vi "FPGASwitch.vi"() -> ()   [LabVIEW 2015]
uses:
  Switch/SwitchStates.ctl
  <vilib>/rvi/eio/common/nirviEmuTemplateMethod_errors.vi
  <vilib>/rvi/Emulation/niFpgaGetClockAttributes.vi
  <vilib>/rvi/Emulation/niFpgaSctlEmulationGetInTimedLoop.vi
  <vilib>/rvi/Emulation/niFpgaEmulationReportErrorSimple.vi
  <vilib>/rvi/Emulation/niFpgaProcessEmulError.vi
  <vilib>/rvi/interface/RandomDataEmulation/nirviRandomDataMultiElementFPGAFIFO.vi
  <instcachedir>/0/nirviRandomDataMultiElementFPGAFIFO_0B1D92D8D7EE43F2AC2E0B59792129FA.lvgen/nirviRandomDataMultiElementFPGAFIFO_0B1D92D8D7EE43F2AC2E0B59792129FA_003.vi
  <vilib>/rvi/interface/RandomDataEmulation/niFpgaRandomDataHandleErrors.vi
  <vilib>/rvi/Emulation/niFpgaCriticalErrorInLSC.vi
  <vilib>/eio/EIONode/EIONode.xnode
  <vilib>/rvi/DataTransferAndStorage/Container/XNode/niFpgaContainer.xnode
  <vilib>/rvi/interface/RandomDataEmulation/nirviRandomDataFpgaMultiElementTemplate.vi
panel:
  out "SwitchState":T1
  in  "stop":bool
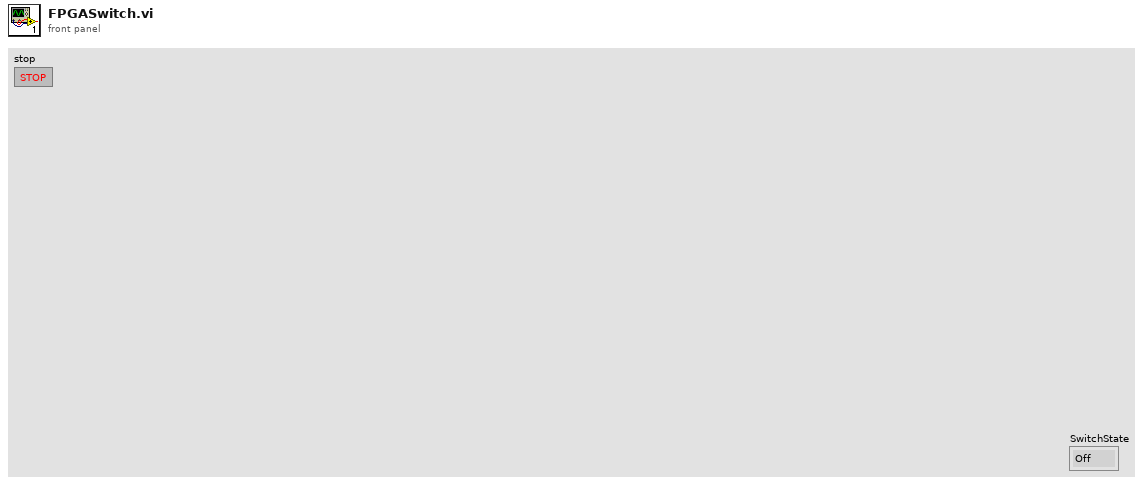
[diagram p1: front panel]
types:
  T1 = typedef "SwitchStates.ctl" = enum16{"Off", "Local", "Remote"}
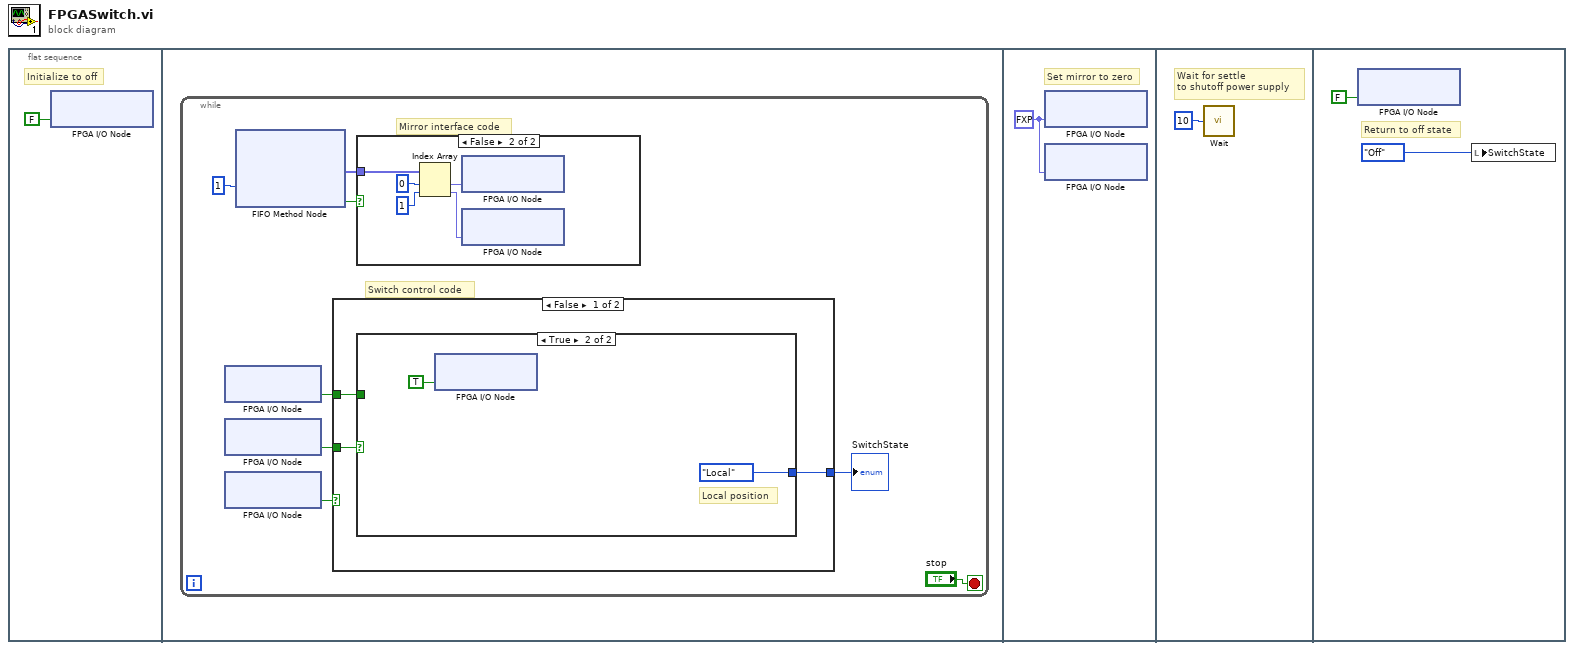
[diagram p0: block diagram]
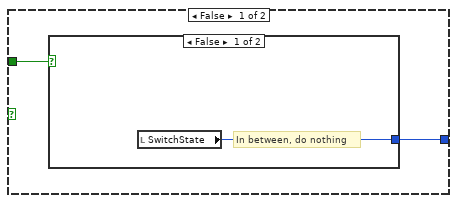
[diagram p3: hidden frame]
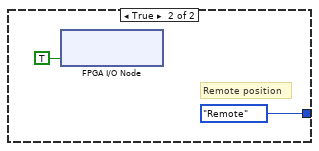
[diagram p4: hidden frame]
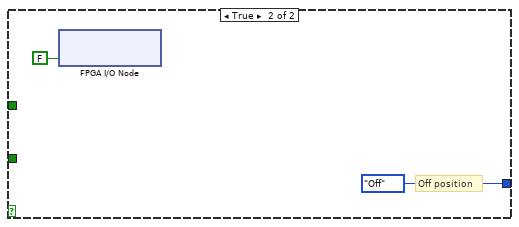
[diagram p5: hidden frame]
diagram:
  n1 = flat-sequence {
    frame #0 {
      # "Initialize to off"
      n2 = xnode "FPGA I/O Node"("Mod6/CH0"=FALSE) -> ()  [unwired: 1 in, 1 out]
    }
    frame #1 {
      n3 = while {
        stop <- "stop" stop-if-true
        # "Switch control code"
        # "Mirror interface code"
        n4 = xnode "FPGA I/O Node"() -> ("Mod7/DI2"=w6:bool)  [unwired: 1 in, 1 out]
        n5 = xnode "FPGA I/O Node"() -> ("Mod7/DI1"=w7:bool)  [unwired: 1 in, 1 out]
        n6 = xnode "FPGA I/O Node"() -> ("Mod7/DI0"=w8:bool)  [unwired: 1 in, 1 out]
        n7 = xnode ("FIFO Method Node")("Timeout"=1) -> ("Element"=w4:fxp<+/-,20,5>[], "Timed Out?"=w2:bool)  [unwired: 1 in, 1 out]
        n8 = case shown="False" w8 {
          tunnel: w7 -> [w17 _]
          tunnel: w6 -> [w16 _]
          tunnel: [w15 SwitchStates."Off" ("SwitchState")] -> w5
          frame False {
            n9 = case shown="True" w17 {
              tunnel: w16 -> [w19 _]
              tunnel: [w18 SwitchStates."Local" ("SwitchState")] -> w15
              frame False {
                n10 = case shown="False" w19 {
                  tunnel: [w20 SwitchStates."Remote" ("SwitchState")] -> w18
                  frame False {
                    # "In between, do nothing"
                    n11 = local read "SwitchState"() -> (w20:T1)
                  }
                  frame True {
                    # "Remote position"
                    n12 = xnode "FPGA I/O Node"("Mod6/CH0"=TRUE) -> ()  [unwired: 1 in, 1 out]
                  }
                }
              }
              frame True {
                # "Local position"
                n13 = xnode "FPGA I/O Node"("Mod6/CH0"=TRUE) -> ()  [unwired: 1 in, 1 out]
              }
            }
          }
          frame True {
            # "Off position"
            n14 = xnode "FPGA I/O Node"("Mod6/CH0"=FALSE) -> ()  [unwired: 1 in, 1 out]
          }
        }
        "SwitchState" <- w5
        n15 = case shown="False" w2 {
          tunnel: w4 -> [_ w14]
          frame True {
          }
          frame False {
            n16 = Index Array(array=w14, index #1=0 ("index"), index #2=1 ("length")) -> (element #1=w11:fxp<+/-,20,5>, element #2=w10:fxp<+/-,20,5>)
            n17 = xnode "FPGA I/O Node"("Mod5/AO2"=w11) -> ()  [unwired: 1 in, 1 out]
            n18 = xnode "FPGA I/O Node"("Mod5/AO3"=w10) -> ()  [unwired: 1 in, 1 out]
          }
        }
      }
    }
    frame #2 {
      w27 = fxp<+/-,20,5> 0.0 ("Mod5/AO2")
      # "Set mirror to zero"
      n19 = xnode "FPGA I/O Node"("Mod5/AO2"=w27) -> ()  [unwired: 1 in, 1 out]
      n20 = xnode "FPGA I/O Node"("Mod5/AO3"=w27) -> ()  [unwired: 1 in, 1 out]
    }
    frame #3 {
      # "Wait for settle \nto shutoff power supply"
      n21 = call "Wait"("Count(mSec)"=u32 10) -> ()  [unwired: 1 out]
    }
    frame #4 {
      # "Return to off state"
      n22 = xnode "FPGA I/O Node"("Mod6/CH0"=FALSE) -> ()  [unwired: 1 in, 1 out]
      n23 = local write "SwitchState"(SwitchStates."Off" ("SwitchState")) -> ()
    }
  }
